vi "004 Crea array temperatures.vi"() -> ()   [LabVIEW 2019]
panel:
  out "output array":dbl[](array[numeric])
  out "Array de tot 10":dbl[](array[numeric])
  out "Array temperatures 80 a -40":dbl[](array[numeric])
  in  "Tamany array \ntemperatures":i32
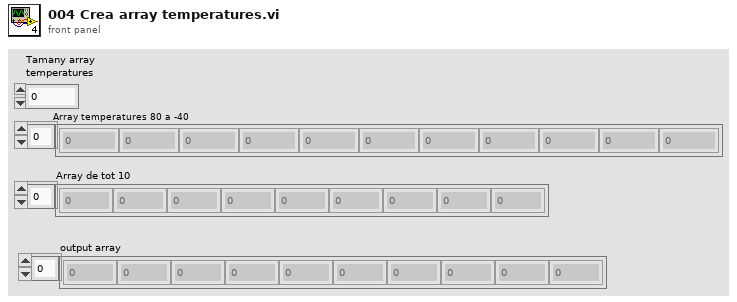
[diagram p1: front panel]
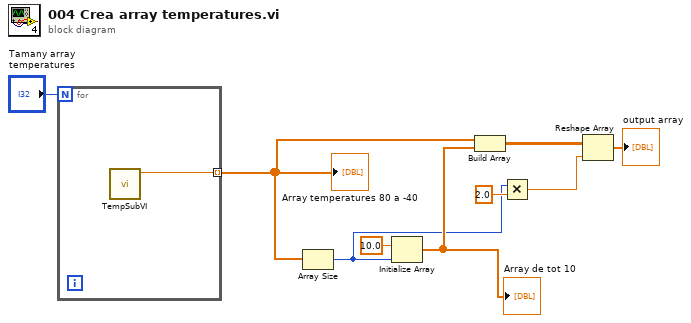
[diagram p0: block diagram]
diagram:
  n1 = for {
    N: "Tamany array \ntemperatures" -> [_]
    tunnel: [w10] -> w7 mode=indexing
    n2 = call "TempSubVI.vi"() -> ("temp"=w10:dbl)  [unwired: 11 in]
  }
  "Array temperatures 80 a -40" <- w7
  n3 = Array Size(array=w7) -> (size(s)=w1:i32)
  n4 = Initialize Array "Initialize Array"(10.0 ("element"), w1) -> (w6:dbl[])
  "Array de tot 10" <- w6
  n5 = Build Array(w7, w6) -> (w5:dbl[][])
  n6 = Multiply(x=w1, y=2.0) -> (x*y=w3:dbl)
  n7 = Reshape Array(w5, w3) -> (→"output array":dbl[])
